vi "加载测试指令.vi"(0 "输入ini文件地址":path=path "F:/Project/GPRS测试/GPRS测试上位机/GPATS.ini", 1 "error in (no error)":errorcluster caption="错误输入（无错误）") -> (2 "加载成功?":bool=TRUE, 3 "指令参数":T1={"测试指令1"={"写参数一"="+TXYBJT GPSQ", "写参数二"="+TXYBJT GPID", "读取版本号"="+TXYBJT GPST", "读取参数一"="+TXYBJT GPCH1", "读取参数二"="+TXYBJT GPCH2", "上电联网"="+TXYBJT GPSM", "指令下线"="+TXYBJT GPSS", "指示灯"=[]}, "测试指令2"={"读取信号强度"="+TXYBJT GPSQ", "读取SIM信息"="+TXYBJT GPID", "读取位置信息"="+TXYBJT GPST", "切换中心参数一"="+TXYBJT GPCH1", "切换中心参数二"="+TXYBJT GPCH2", "强制短信一"="+TXYBJT GPSM", "强制短信二"="+TXYBJT GPSS", "指示灯"=[]}, "等待时间"=[], "校验字符"=[], "GPRS参数"={"GPRS参数一"="", "GPRS参数二"=""}}, 4 "error out":errorcluster caption="错误输出")   [LabVIEW 2015]
uses:
  <vilib>/Utility/config.llb/Read Key (String).vi
  <vilib>/Utility/config.llb/Read Key (U32).vi
  <vilib>/Utility/config.llb/NI_LVConfig.lvlib
panel:
  # "TER   TCP  UDP  SMS"
  # "TER   TCP  UDP  SMS"
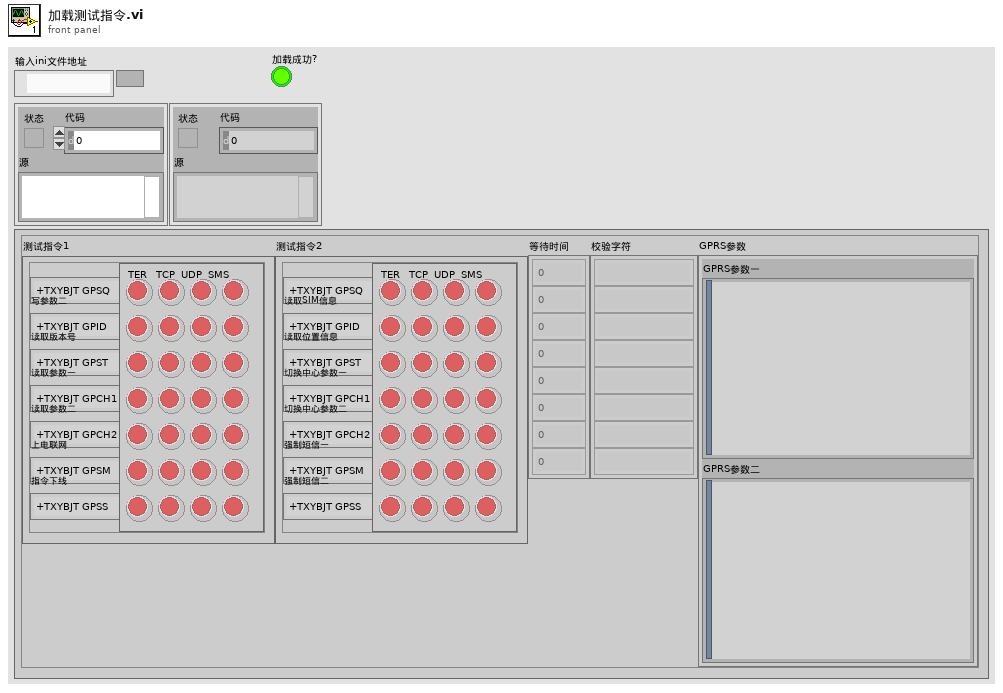
[diagram p1: front panel]
types:
  T1 = typedef "初始化测试指令.ctl" = cluster{"测试指令1":T2, "测试指令2":T3, "等待时间":u32[], "校验字符":string[], "GPRS参数":T4}
  T2 = typedef "指令参数1.ctl" = cluster{"写参数一":string, "写参数二":string, "读取版本号":string, "读取参数一":string, "读取参数二":string, "上电联网":string, "指令下线":string, "指示灯":bool[][]}
  T3 = typedef "指令参数2.ctl" = cluster{"读取信号强度":string, "读取SIM信息":string, "读取位置信息":string, "切换中心参数一":string, "切换中心参数二":string, "强制短信一":string, "强制短信二":string, "指示灯":bool[][]}
  T4 = typedef "GPRS参数.ctl" = cluster{"GPRS参数一":string, "GPRS参数二":string}
  T5 = typedef "NI_LVConfig.lvlib/Config Data RefNum.ctl" = refnum<k1>
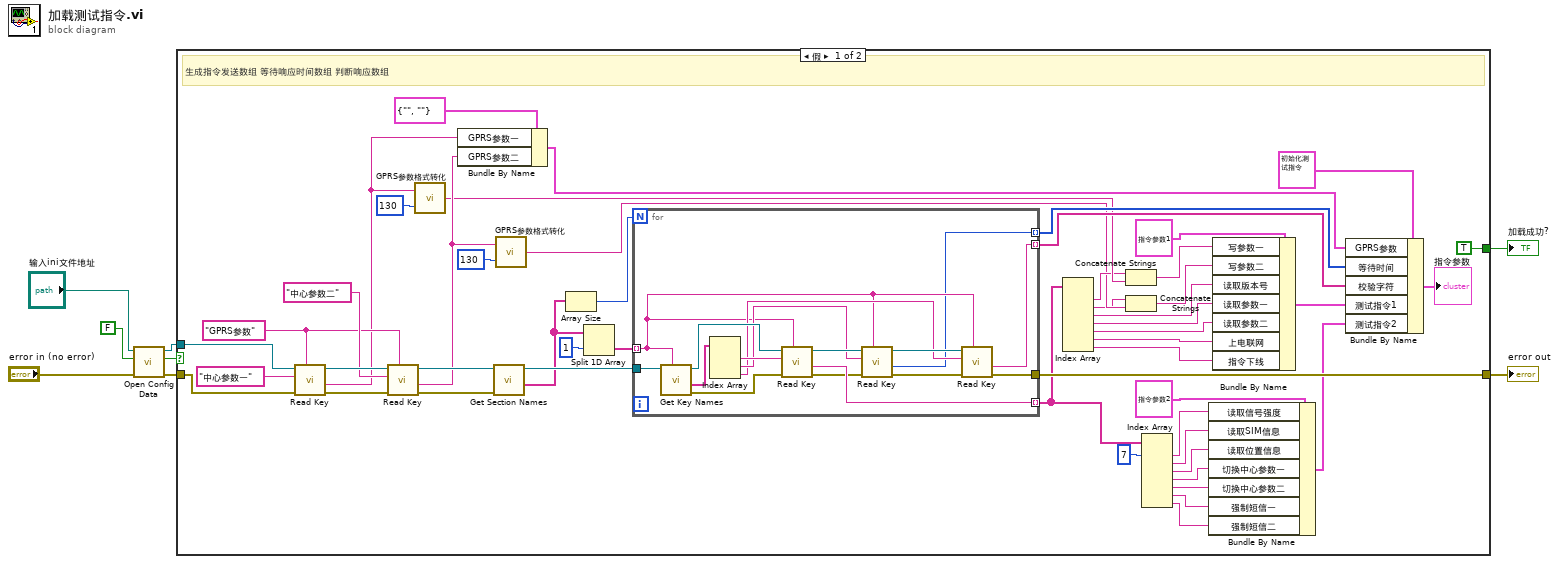
[diagram p0: block diagram]
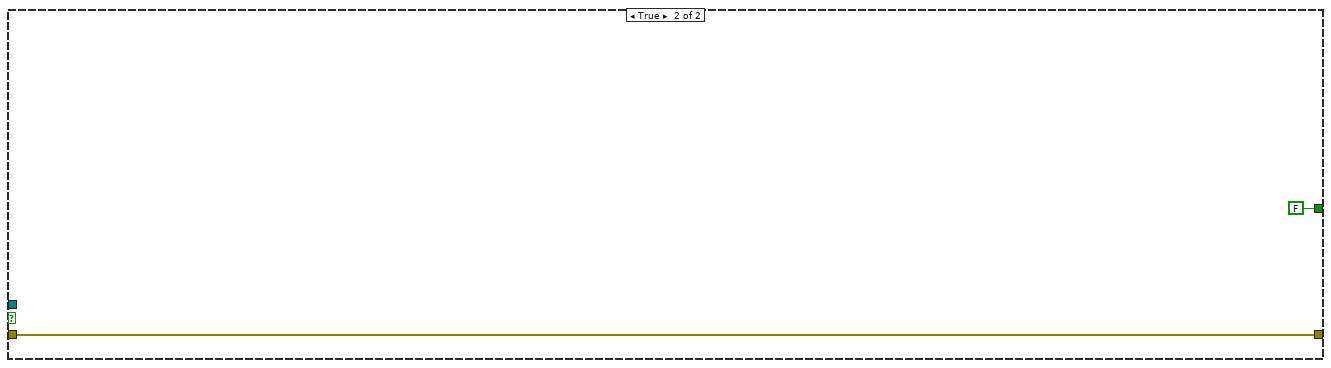
[diagram p2: hidden frame]
diagram:
  n1 = call <vilib>:"Open Config Data.vi"("error in (no error)"="error in (no error)", "create file if necessary (T)"=FALSE, "configuration file path"="输入ini文件地址") -> ("error out"=w8:errorcluster, "file created?"=w4:bool, "refnum"=w5:T5)  [unwired: 6 in]
  n2 = case shown="假" w4 {
    tunnel: w8 -> [w27 w75]
    tunnel: w5 -> [w29 _]
    tunnel: [TRUE FALSE] -> w3
    tunnel: [w55 w75] -> w1
    frame False {
      w30 = "GPRS参数" ("key")
      # "生成指令发送数组 等待响应时间数组 判断响应数组"
      n3 = call-poly <vilib>:"Read Key.vi"("section"=w30, "error in (no error)"=w27, "key"="中心参数一", "refnum"=w29) -> ("error out"=w31:errorcluster, "value"=w23:string, "refnum out"=w33:T5)  [unwired: 4 in, 1 out]
      n4 = call-poly <vilib>:"Read Key.vi"("section"=w30, "error in (no error)"=w31, "key"="中心参数二", "refnum"=w33) -> ("error out"=w26:errorcluster, "value"=w20:string, "refnum out"=w28:T5)  [unwired: 4 in, 1 out]
      n5 = call "GPRS参数格式转化.vi"("参数大小"=u16 130, "参数字符串(十进制)"=w23) -> ("参数字符串(十六进制)"=w19:string)
      n6 = Bundle By Name(cluster=T4 {"GPRS参数一"="", "GPRS参数二"=""} ("参数"), "GPRS参数一"=w23, "GPRS参数二"=w20) -> (w24:T4)
      n7 = call <vilib>:"Get Section Names.vi"("error in (no error)"=w26, "refnum"=w28) -> ("section names"=w13:string[], "refnum out"=w56:T5)  [unwired: 7 in, 1 out]
      n8 = call "GPRS参数格式转化.vi"("参数大小"=u16 130, "参数字符串(十进制)"=w20) -> ("参数字符串(十六进制)"=w16:string)
      n9 = Array Size(array=w13) -> (size(s)=w57:i32)
      n10 = Split 1D Array(array=w13, index=1 ("索引")) -> (second subarray=w11:string[])  [unwired: 1 out]
      n11 = for {
        N: w57 -> [_]
        tunnel: w11 -> [w65] mode=indexing
        tunnel: w56 -> [w73]
        tunnel: [w64] -> w53 mode=indexing
        tunnel: [w63] -> w54 mode=indexing
        tunnel: [w62] -> w35 mode=indexing
        tunnel: [w59] -> w55
        n12 = call <vilib>:"Get Key Names.vi"("section"=w65, "refnum"=w73) -> ("error out"=w74:errorcluster, "key names"=w69:string[], "refnum out"=w72:T5)  [unwired: 6 in, 1 out]
        n13 = Index Array(array=w69) -> (element #1=w68:string, element #2=w67:string, element #3=w66:string)  [unwired: 3 in]
        n14 = call-poly <vilib>:"Read Key.vi"("section"=w65, "error in (no error)"=w74, "key"=w68, "refnum"=w72) -> ("error out"=w61:errorcluster, "value"=w62:string, "refnum out"=w70:T5)  [unwired: 4 in, 1 out]
        n15 = call-poly <vilib>:"Read Key.vi"("section"=w65, "error in (no error)"=w61, "key"=w67, "refnum"=w70) -> ("error out"=w60:errorcluster, "value"=w63:u32, "refnum out"=w71:T5)  [unwired: 4 in, 1 out]
        n16 = call-poly <vilib>:"Read Key.vi"("section"=w65, "error in (no error)"=w60, "key"=w66, "refnum"=w71) -> ("error out"=w59:errorcluster, "value"=w64:string)  [unwired: 4 in, 2 out]
      }
      n17 = Index Array(array=w35) -> (element #1=w18:string, element #2=w14:string, element #3=w38:string, element #4=w39:string, element #5=w40:string, element #6=w41:string, element #7=w42:string)  [unwired: 7 in]
      n18 = Concatenate Strings(w18, w19) -> (w17:string)
      n19 = Concatenate Strings(w14, w16) -> (w15:string)
      n20 = Index Array(array=w35, index #1=7 ("索引")) -> (element #1=w45:string, element #2=w46:string, element #3=w50:string, element #4=w51:string, element #5=w52:string, element #6=w47:string, element #7=w48:string)  [unwired: 6 in]
      n21 = Bundle By Name(cluster=T3 {"读取信号强度"="+TXYBJT GPSQ", "读取SIM信息"="+TXYBJT GPID", "读取位置信息"="+TXYBJT GPST", "切换中心参数一"="+TXYBJT GPCH1", "切换中心参数二"="+TXYBJT GPCH2", "强制短信一"="+TXYBJT GPSM", "强制短信二"="+TXYBJT GPSS", "指示灯"=[[FALSE, FALSE, FALSE, FALSE], [FALSE, FALSE, FALSE, FALSE], [FALSE, FALSE, FALSE, FALSE], [FALSE, FALSE, FALSE, FALSE], [FALSE, FALSE, FALSE, FALSE], [FALSE, FALSE, FALSE, FALSE], [FALSE, FALSE, FALSE, FALSE]]} ("测试指令2常量"), "读取信号强度"=w45, "读取SIM信息"=w46, "读取位置信息"=w50, "切换中心参数一"=w51, "切换中心参数二"=w52, "强制短信一"=w47, "强制短信二"=w48) -> (w37:T3)
      n22 = Bundle By Name(cluster=T2 {"写参数一"="+TXYBJT GPSQ", "写参数二"="+TXYBJT GPID ", "读取版本号"="+TXYBJT GPST", "读取参数一"="+TXYBJT GPCH1", "读取参数二"="+TXYBJT GPCH2", "上电联网"="+TXYBJT GPSM", "指令下线"="+TXYBJT GPSS", "指示灯"=[[FALSE, FALSE, FALSE, FALSE], [FALSE, FALSE, FALSE, FALSE], [FALSE, FALSE, FALSE, FALSE], [FALSE, FALSE, FALSE, FALSE], [FALSE, FALSE, FALSE, FALSE], [FALSE, FALSE, FALSE, FALSE], [FALSE, FALSE, FALSE, FALSE]]} ("测试指令1常量"), "写参数一"=w17, "写参数二"=w15, "读取版本号"=w38, "读取参数一"=w39, "读取参数二"=w40, "上电联网"=w41, "指令下线"=w42) -> (w36:T2)
      n23 = Bundle By Name(cluster=T1 {"测试指令1"={"写参数一"="+TXYBJT GPSQ", "写参数二"="+TXYBJT GPID", "读取版本号"="+TXYBJT GPST", "读取参数一"="+TXYBJT GPCH1", "读取参数二"="+TXYBJT GPCH2", "上电联网"="+TXYBJT GPSM", "指令下线"="+TXYBJT GPSS", "指示灯"=[]}, "测试指令2"={"读取信号强度"="+TXYBJT GPSQ", "读取SIM信息"="+TXYBJT GPID", "读取位置信息"="+TXYBJT GPST", "切换中心参数一"="+TXYBJT GPCH1", "切换中心参数二"="+TXYBJT GPCH2", "强制短信一"="+TXYBJT GPSM", "强制短信二"="+TXYBJT GPSS", "指示灯"=[]}, "等待时间"=[], "校验字符"=[], "GPRS参数"={"GPRS参数一"="", "GPRS参数二"=""}} ("指令参数"), "GPRS参数"=w24, "等待时间"=w54, "校验字符"=w53, "测试指令1"=w36, "测试指令2"=w37) -> (→"指令参数":T1)
    }
    frame True {
    }
  }
  "加载成功?" <- w3
  "error out" <- w1
